vi "RT_Aceleration in DLR Navigation Reference System(SubVI).vi"(5 "i":i32, 6 "dt(s)":dbl, 7 "Data":dbl[][](array[numeric]), 8 "Fco (N)":dbl[](array[numeric]), 9 "FA":dbl[](array[numeric]), 10 "FG":dbl[](array[numeric]), 11 "FE":dbl[](array[numeric])) -> (3 "acc":dbl[](array[numeric]))   [LabVIEW 2017]
uses:
  <vilib>/Analysis/_algsub.llb/Vector Norm Type.ctl
  <vilib>/Analysis/_algsub.llb/Real Vector Norm.vi
  <vilib>/Analysis/NI_AALPro.lvlib
panel:
  out "M":dbl
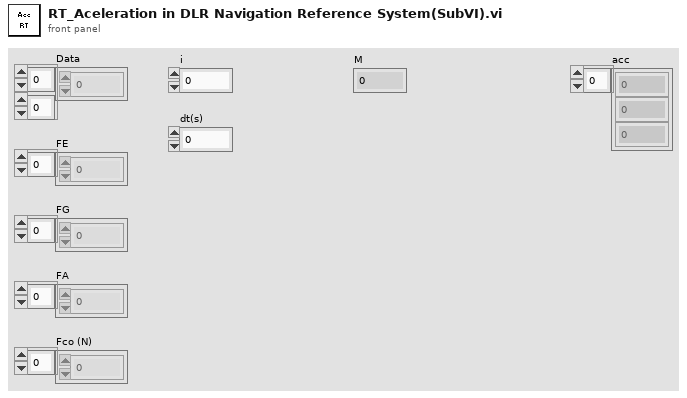
[diagram p1: front panel]
types:
  T1 = typedef "NI_AALPro.lvlib/Vector Norm Type.ctl" = u16
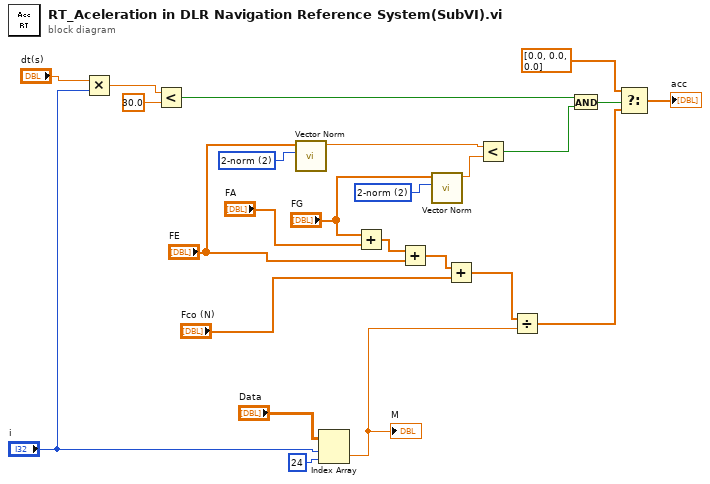
[diagram p0: block diagram]
diagram:
  w9 = T1 2 items=["1-norm"=1, "2-norm"=2, "Inf-norm"=3, "-Inf-norm"=4, "User Defined"=5] ("norm type")
  w11 = T1 2 items=["1-norm"=1, "2-norm"=2, "Inf-norm"=3, "-Inf-norm"=4, "User Defined"=5] ("norm type")
  n1 = Multiply(x="dt(s)", y="i") -> (x*y=w14:dbl)
  n2 = Less?(x=w14, y=30.0) -> (x < y?=w12:bool)
  n3 = call-poly <vilib>:"Vector Norm.vi"("norm type"=w11, "Input Vector"="FE") -> ("norm"=w7:dbl)  [unwired: 8 in, 1 out]
  n4 = Index Array(array="Data", index (row)="i", index (col)=24 ("disabled index (col)")) -> (element=w24:dbl)
  "M" <- w24
  n5 = Add(x="FG", y="FA") -> (x+y=w19:dbl[])
  n6 = Add(x=w19, y="FE") -> (x+y=w20:dbl[])
  n7 = call-poly <vilib>:"Vector Norm.vi"("norm type"=w9, "Input Vector"="FG") -> ("norm"=w6:dbl)  [unwired: 8 in, 1 out]
  n8 = Add(x=w20, y="Fco (N)") -> (x+y=w23:dbl[])
  n9 = Less?(x=w7, y=w6) -> (x < y?=w5:bool)
  n10 = Divide(x=w23, y=w24) -> (x/y=w3:dbl[])
  n11 = And(x=w12, y=w5) -> (x .and. y?=w4:bool)
  n12 = Select(t=dbl[] [0.0, 0.0, 0.0], s=w4, f=w3) -> (s? t:f=→"acc":dbl[])
